vi "Parallelism.vi"() -> ()   [LabVIEW 2014]
panel:
  out "error out":errorcluster
  in  "error in (no error)":errorcluster
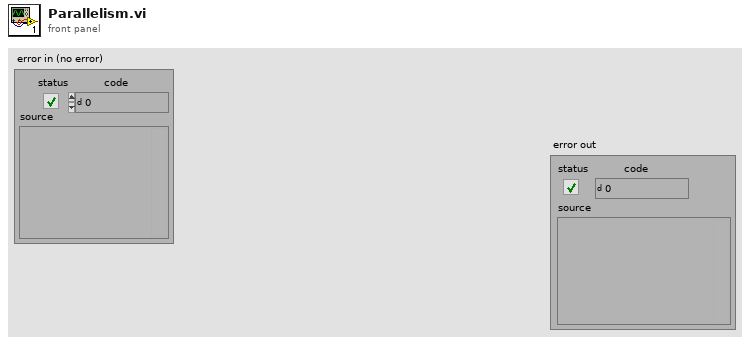
[diagram p1: front panel]
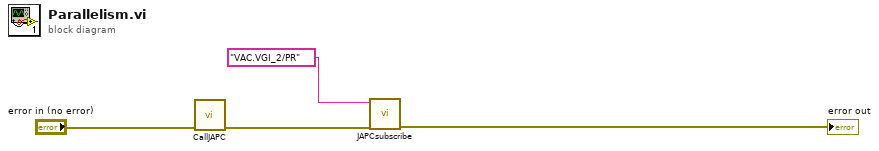
[diagram p0: block diagram]
diagram:
  n1 = call "CallJAPC.vi"("error in"="error in (no error)") -> ("error out"=w1:errorcluster)  [unwired: 10 in]
  n2 = call "JAPCsubscribe.vi"("error in (no error)"=w1, "URL"="VAC.VGI_2/PR") -> ("error out"=→"error out":errorcluster)  [unwired: 9 in]
